vi "InitDLLs.vi"(0 "scenarios2VirtPlantOutputMsgs":refnum<vi>, 1 "scenarios2VerifierOutputMsgs":refnum<vi>, 2 "algOutputMsgs":refnum<vi>, 3 "verifier2GUIOutputMsgs":refnum<vi>, 4 "virtualPlant2GUIOutputMsgs":refnum<vi>, 5 "algStates":refnum<vi>, 6 "scenarios2AlgOutputMsgs":refnum<vi>, 7 "vplantStates":refnum<vi>, 8 "algOutputPorts":refnum<vi>, 9 "verStates":refnum<vi>, 10 "algInputPorts":refnum<vi>, 11 "scenarioStates":refnum<vi>, 18 "verifier2scenariousControlOutMsgs":refnum<vi>) -> ()   [LabVIEW 2010]
uses:
  DLL-s/MakeFullImmitationStepDLL/Release/MakeFullImmitationStepDLL.dll
panel:
  out "Value":cluster{"TimeInState":u16, "cur_state":i8}[](array[cluster])
  out "return type":i32
  out "Load NEW DLLs error":i32
  out "Init error":i32
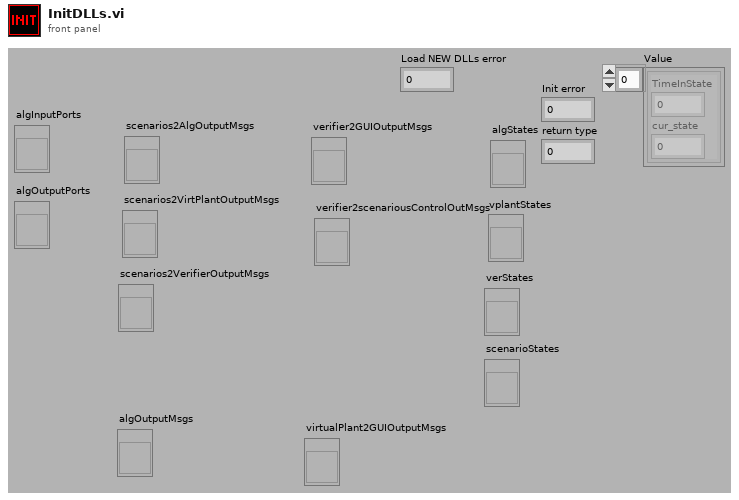
[diagram p1: front panel]
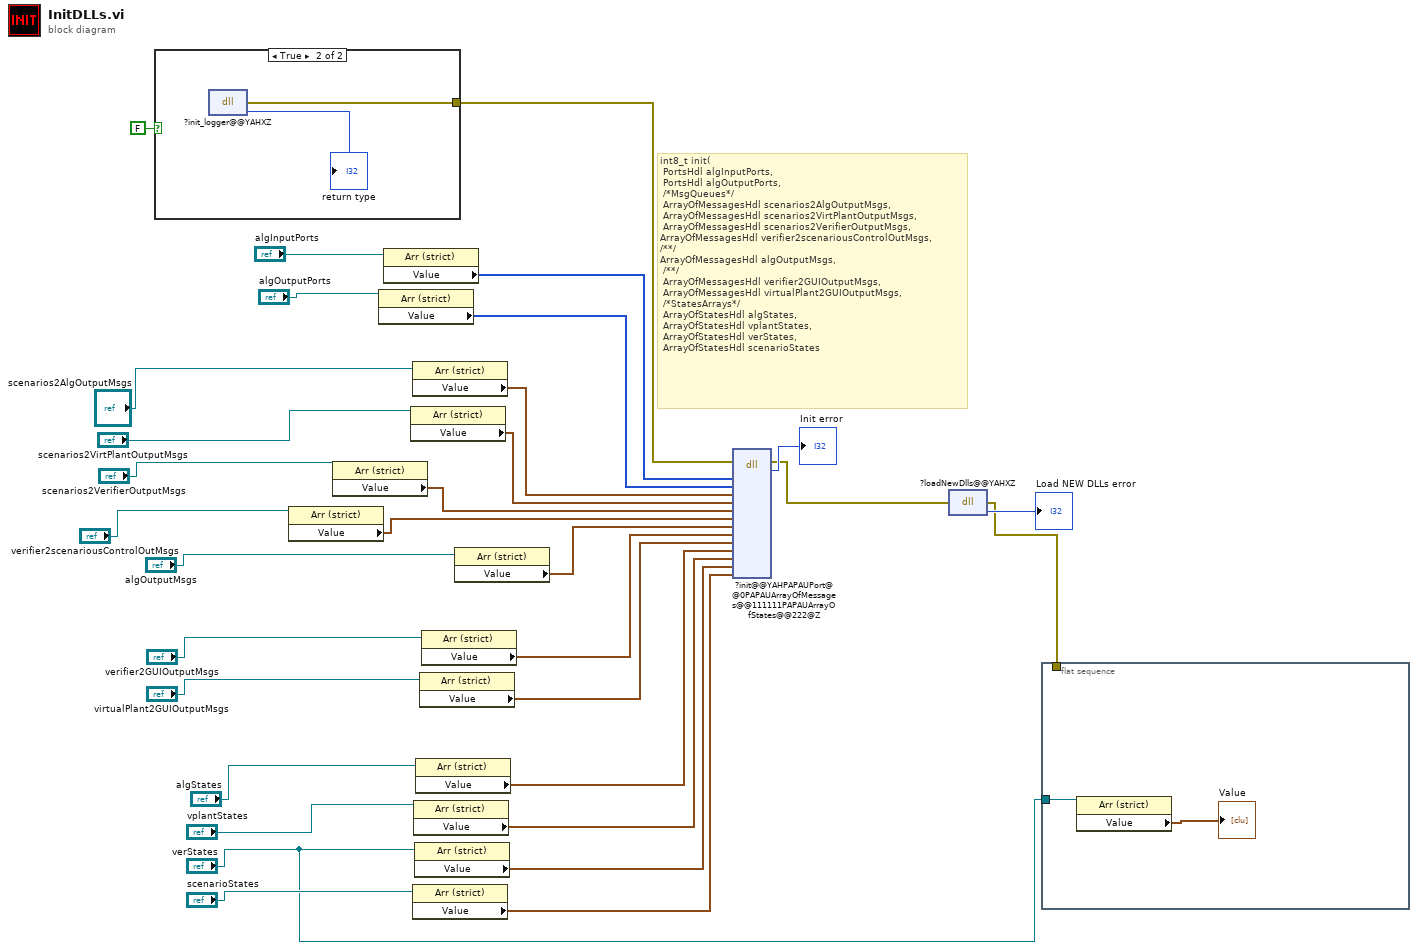
[diagram p0: block diagram]
diagram:
  # "int8_t init(\n\tPortsHdl algInputPorts,\n\tPortsHdl algOutputPorts,\n\t/*MsgQueues*/\n\tArrayOfMessagesHdl scenarios2AlgOutputMsgs,\n\tArrayOfMessagesHdl scenarios2VirtPlantOutputMsgs,\n\tArrayOfMessagesHdl scenarios2VerifierOutputMsgs,\nArrayOfMessagesHdl verifier2scenariousControlOutMsgs,\n/**/\t\nArrayOfMessagesHdl algOutputMsgs,\n\t/**/\n\tArrayOfMessagesHdl verifier2GUIOutputMsgs,\n\tArrayOfMessagesHdl virtualPlant2GUIOutputMsgs,\n\t/*StatesArrays*/\n\tArrayOfStatesHdl algStates,\n\tArrayOfStatesHdl vplantStates,\n\tArrayOfStatesHdl verStates,\n\tArrayOfStatesHdl scenarioStates"
  n1 = case shown="True" FALSE {
    tunnel: [_ w34] -> w4
    frame False {
    }
    frame True {
      n2 = dll-call lib="D:/Liakh Tanya/Dissertation/Complex/DLL-s/MakeFullImmitationStepDLL/Release/MakeFullImmitationStepDLL.dll" fn="?init_logger@@YAHXZ" label="init_logger@@YAHXZ"() -> (error out=w34:errorcluster, "return type"=→"return type":i32)  [unwired: 3 in, 1 out]
    }
  }
  n3 = property class="Arr (strict)"(reference="verifier2scenariousControlOutMsgs") -> ("Value"=w7:cluster{"MSG":i16, "param":i32, "Type":i16}[])  [unwired: 1 in, 2 out]
  n4 = property class="Arr (strict)"(reference="scenarios2VerifierOutputMsgs") -> ("Value"=w22:cluster{"MSG":i16, "param":i32, "Type":i16}[])  [unwired: 1 in, 2 out]
  n5 = property class="Arr (strict)"(reference="algOutputPorts") -> ("Value"=w25:i8[])  [unwired: 1 in, 2 out]
  n6 = property class="Arr (strict)"(reference="algInputPorts") -> ("Value"=w26:i8[])  [unwired: 1 in, 2 out]
  n7 = property class="Arr (strict)"(reference="scenarios2VirtPlantOutputMsgs") -> ("Value"=w23:cluster{"MSG":i16, "param":i32, "Type":i16}[])  [unwired: 1 in, 2 out]
  n8 = property class="Arr (strict)"(reference="scenarios2AlgOutputMsgs") -> ("Value"=w24:cluster{"MSG":i16, "param":i32, "Type":i16}[])  [unwired: 1 in, 2 out]
  n9 = property class="Arr (strict)"(reference="scenarioStates") -> ("Value"=w10:cluster{"TimeInState":u16, "cur_state":i8}[])  [unwired: 1 in, 2 out]
  n10 = property class="Arr (strict)"(reference="vplantStates") -> ("Value"=w12:cluster{"TimeInState":u16, "cur_state":i8}[])  [unwired: 1 in, 2 out]
  n11 = property class="Arr (strict)"(reference="verStates") -> ("Value"=w11:cluster{"TimeInState":u16, "cur_state":i8}[])  [unwired: 1 in, 2 out]
  n12 = property class="Arr (strict)"(reference="algStates") -> ("Value"=w13:cluster{"TimeInState":u16, "cur_state":i8}[])  [unwired: 1 in, 2 out]
  n13 = property class="Arr (strict)"(reference="virtualPlant2GUIOutputMsgs") -> ("Value"=w17:cluster{"MSG":i16, "param":i32, "Type":i16}[])  [unwired: 1 in, 2 out]
  n14 = property class="Arr (strict)"(reference="verifier2GUIOutputMsgs") -> ("Value"=w18:cluster{"MSG":i16, "param":i32, "Type":i16}[])  [unwired: 1 in, 2 out]
  n15 = property class="Arr (strict)"(reference="algOutputMsgs") -> ("Value"=w21:cluster{"MSG":i16, "param":i32, "Type":i16}[])  [unwired: 1 in, 2 out]
  n16 = dll-call lib="D:/Liakh Tanya/Dissertation/Complex/DLL-s/MakeFullImmitationStepDLL/Release/MakeFullImmitationStepDLL.dll" fn="?init@@YAHPAPAUPort@@0PAPAUArrayOfMessages@@111111PAPAUArrayOfStates@@222@Z" label="Init"(error in=w4, "algInputPorts"=w26, "algOutputPorts"=w25, "scenarios2AlgOutputMsgs"=w24, "scenarios2VirtPlantOutputMsgs"=w23, "scenarios2VerifierOutputMsgs"=w22, "verifier2scenariousControlOutMsgs,"=w7, "algOutputMsgs"=w21, "verifier2GUIOutputMsgs"=w18, "virtualPlant2GUIOutputMsgs"=w17, "algStates"=w13, "vplantStates"=w12, "verStates"=w11, "scenarioStates"=w10) -> (error out=w6:errorcluster, "error"=→"Init error":i32)  [unwired: 15 in, 1 out]
  n17 = dll-call lib="D:/Liakh Tanya/Dissertation/Complex/DLL-s/MakeFullImmitationStepDLL/Release/MakeFullImmitationStepDLL.dll" fn="?loadNewDlls@@YAHXZ" label="Load NEW DLLs"(error in=w6) -> (error out=w2:errorcluster, "error"=→"Load NEW DLLs error":i32)  [unwired: 2 in, 1 out]
  n18 = flat-sequence {
    tunnel: w2 -> [_]
    tunnel: "verStates" -> [w36]
    frame #0 {
      n19 = property class="Arr (strict)"(reference=w36) -> ("Value"=→"Value":cluster{"TimeInState":u16, "cur_state":i8}[])  [unwired: 1 in, 2 out]
    }
  }
